vi "SoftFrontPanel.vi"(8 "error in (no error)":errorcluster, 11 "ACIR Instrument":refnum<class "ACIR Instrument.lvclass">) -> (0 "error out":errorcluster, 3 "ACIR Instrument out":refnum<class "ACIR Instrument.lvclass">)   [LabVIEW 2025, in "ACIR.lvlib" / "ACIR Instrument.lvclass"]
doc: "Copyright 2017 National Instruments Corporation\n\nLicensed under the Apache License, Version 2.0 (the \"License\"); you may not use this file except in compliance with the License. You may obtain a copy of the License at http://www.apache.org/licenses/LICENSE-2.0\nUnless required by applicable law or agreed to in writing, software distributed under the License is distributed on an \"AS IS\" BASIS, WITHOUT WARRANTIES OR CONDITIONS OF ANY KIND, either express or implied. See the License for the specific language governing permissions and limitations under the License."
uses:
  ACIR Instrument.lvclass
  ACIR Instrument.lvclass/ACIR Instrument.ctl
  Users/Public/Documents/Sandia National Labs/TSS Plugin/CEF.lvlibp
  ACIR configuration/ACIR configuration.lvclass
panel:
  out "SFP":cluster{"Data":dbl, "Chname":string}={"Data"=0.0, "Chname"="Ch0"}
  out "Instrument":string caption="Instrument ::"
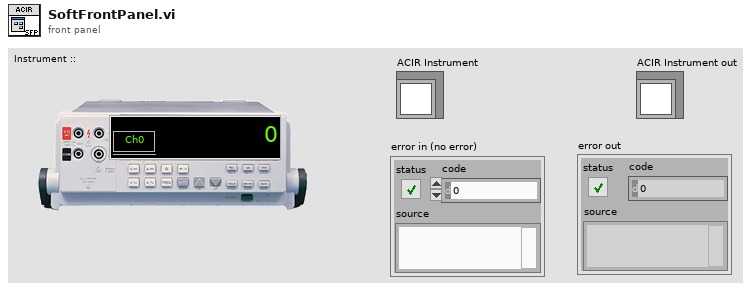
[diagram p1: front panel]
types:
  T1 = enum32{"Invalid", "Default", "Floating", "Floating/Auto-Hide", "Modal"}
  T2 = typedef "Abstract Engine.lvlibp/Instrument configuration.lvclass/Default Instrument.ctl" = cluster{"Type":string, "Address":string, "SW Alias":string, "Description":string, "Enabled":bool}
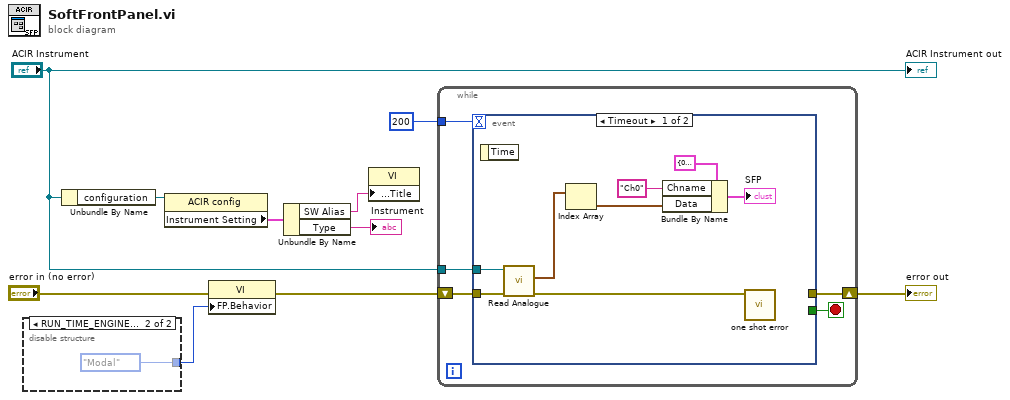
[diagram p0: block diagram]
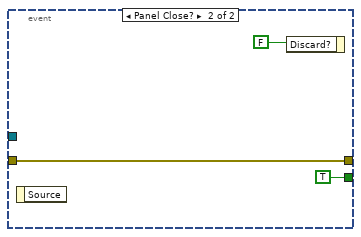
[diagram p2: hidden frame]
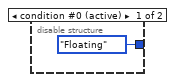
[diagram p3: hidden frame]
diagram:
  n1 = disable-structure shown="RUN_TIME_ENGINE==True" {
    disable-tunnel: [T1."Floating" ("Front Panel Window:Behavior") T1."Modal" ("Front Panel Window:Behavior")] -> w9
    frame condition #0 (active) {
    }
    frame condition #1 {
    }
  }
  n2 = Unbundle By Name("ACIR Instrument") -> ("configuration"=w6:refnum<class "ACIR configuration.lvclass">)
  n3 = property class="ACIR config"(reference=w6) -> ("Instrument Setting"=w5:T2)  [unwired: 1 in, 2 out]
  n4 = property class="VI"(error in="error in (no error)", "FP.Behavior"=w9) -> (error out=w7:errorcluster)  [unwired: 1 in, 1 out]
  n5 = Unbundle By Name(w5) -> ("SW Alias"=w3:string, "Type"=→"Instrument":string)
  n6 = property class="VI"("Front Panel.Title"=w3) -> ()  [unwired: 2 in, 2 out]
  n7 = while {
    shift-right: [w15] -> w1
    shift-left: w7 -> [w16]
    tunnel: "ACIR Instrument" -> [w14]
    tunnel: 200 -> [w13]
    stop <- w17 stop-if-true
    n8 = event shown="[0] Timeout" {
      selector: _ -> [_ _]
      dyn-events: _ -> [_ _]
      timeout: w13 -> [_ _]
      tunnel: [_ TRUE] -> w17
      tunnel: [_ w26] -> w15
      tunnel: w16 -> [w21 w26]
      tunnel: w14 -> [w20 _]
      event Timeout {
        n9 = event-data() -> ()  [unwired: 1 in, 1 out]
        n10 = call-dynamic "Read Analogue.vi"("error in (no error)"=w21, "ACIR Instrument"=w20) -> ("error out"=w19:errorcluster, "Waveforms"=w18:waveform(dbl)[])  [unwired: 7 in, 1 out]
        n11 = Index Array(array=w18) -> (element=w22:waveform(dbl))  [unwired: 1 in]
        n12 = Bundle By Name(cluster=cluster{"Data":dbl, "Chname":string} {"Data"=0.0, "Chname"="Ch0"} ("SFP"), "Chname"="Ch0", "Data"=w22) -> (→"SFP":cluster{"Data":dbl, "Chname":string})
        n13 = call "one shot error.vi"("error in"=w19) -> ()  [unwired: 11 in]
      }
      event Panel Close? {
        n14 = event-data() -> ()  [unwired: 1 in, 1 out]
        n15 = event-data("Discard?"=FALSE) -> ()  [unwired: 1 in, 1 out]
      }
    }
  }
  "error out" <- w1
  "ACIR Instrument out" <- "ACIR Instrument"
